vi "sensors mega.vi"() -> ()   [LabVIEW 2011]
uses:
  <vilib>/LabVIEW Interface for Arduino/Type Defs/Board Type.ctl
  <vilib>/LabVIEW Interface for Arduino/Type Defs/Pin Mode.ctl
  <vilib>/LabVIEW Interface for Arduino/Type Defs/Analog Pin.ctl
  <vilib>/LabVIEW Interface for Arduino/LabVIEW Interface for Arduino.lvlib
panel:
  in  "stop 12":bool
  out "Voltage 3":dbl(knob) scale=0.0..5.0
  out "tank":dbl(slide) scale=0.0..100.0
  out "Voltage 2":dbl(knob) scale=0.0..5.0
  out "Voltage":dbl(knob) scale=0.0..5.0
  in  "stop 11":bool
  out "Light Pos1":dbl(slide) scale=0.0..100.0
  out "Light Pos2":dbl(slide) scale=0.0..100.0
  out "Solar Pos1":bool
  out "Solar Pos2":bool
  in  "stop 10":bool
  out "Month":dbl
  in  "stop 8":bool
  in  "Wahsing Machine":bool
  in  "Dryer":bool
  in  "stop 7":bool
  in  "stop 6":bool
  in  "stop":bool
  out "Light Intensity (0 - 100) Pos2":dbl(knob) scale=0.0..100.0
  in  "stop 3":bool
  in  "stop 9":bool
  out "Water Voltage":dbl(knob) scale=0.0..5.0
  out "Low Level Water":bool
  in  "Units 2":enum16{"Celsius", "Fahrenheit", "Kelvin"}(ring)
  in  "stop 5":bool
  out "Water Temperature":dbl(slide) scale=0.0..100.0
  in  "Units":enum16{"Celsius", "Fahrenheit", "Kelvin"}(ring)
  in  "stop 4":bool
  out "Temperature Inside":dbl(slide) scale=0.0..100.0
  out "Light Intensity (0 - 100)Pos 1":dbl(knob) scale=0.0..100.0
  in  "stop 2":bool
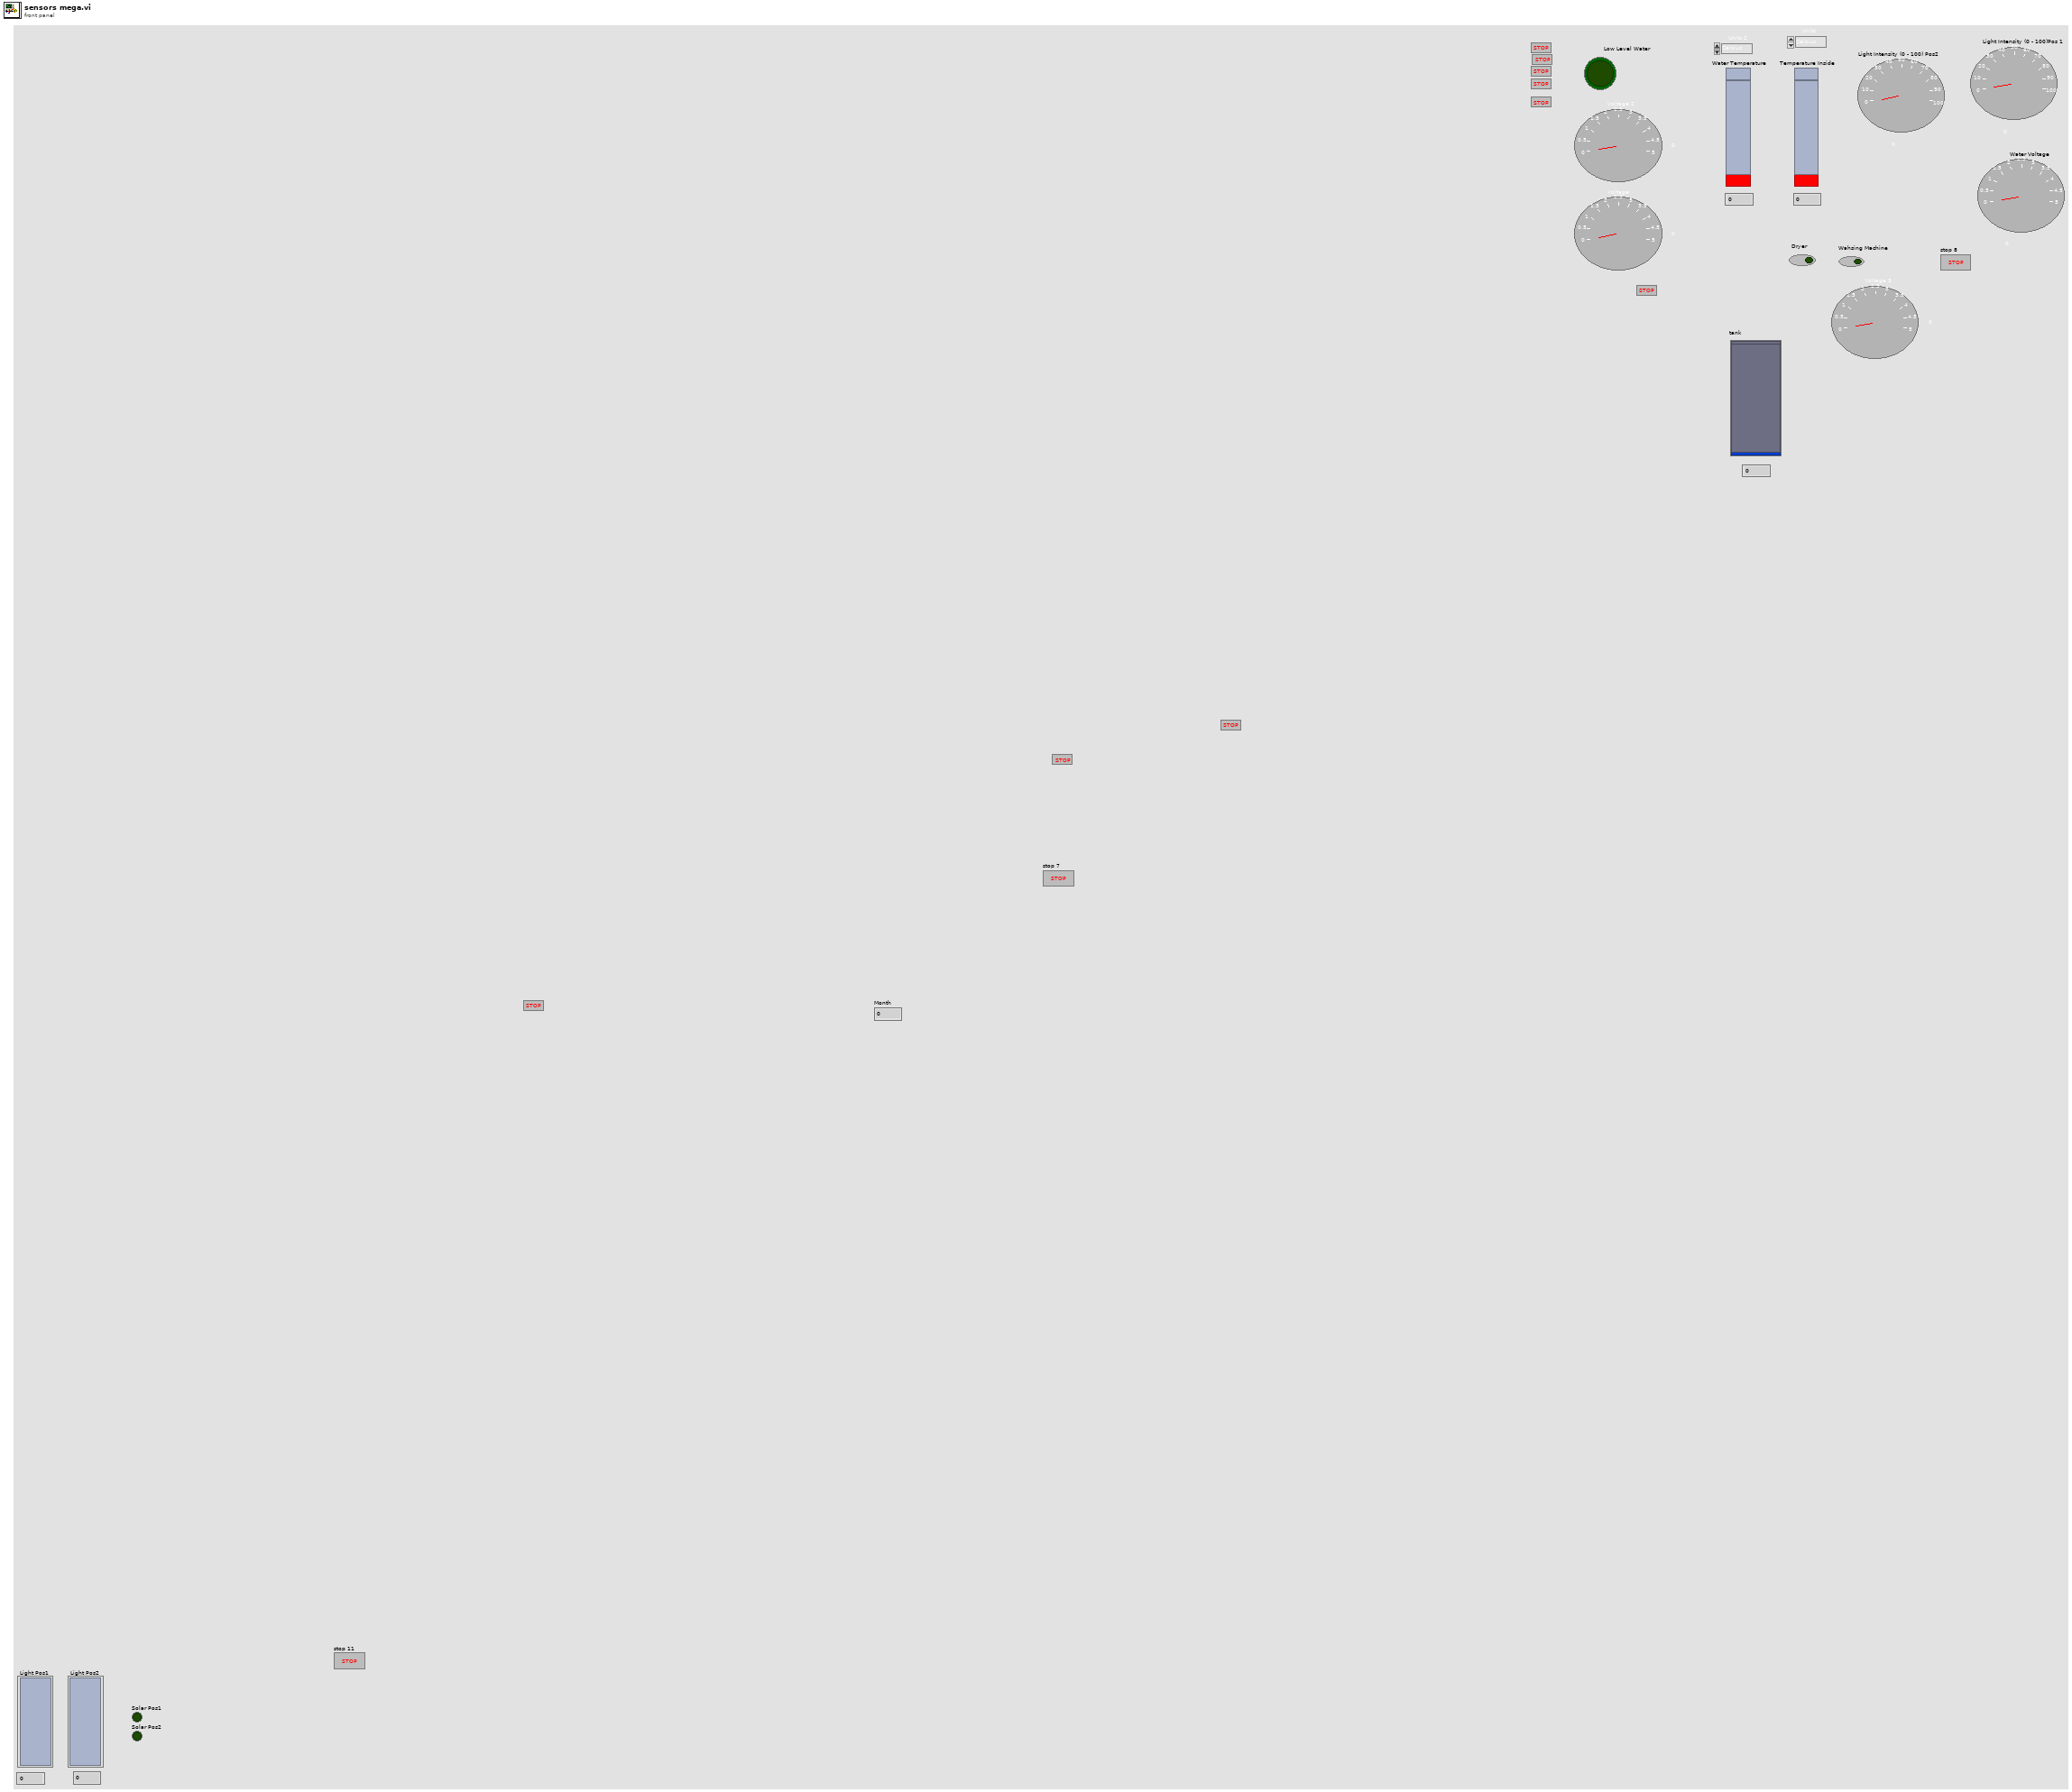
[diagram p1: front panel]
types:
  T1 = typedef "LabVIEW Interface for Arduino.lvlib/Board Type.ctl" = enum16{"Uno", "Dimuelanove w/Atmega 328", "Mega 2560"}
  T2 = typedef "LabVIEW Interface for Arduino.lvlib/Arduino Resource.ctl" = cluster{"VISA resource":refnum<visa-resource-name>, "Board Type":T1, "Connection Type":enum8{"USB / Serial"}, "Bytes Per Packet (15)":u8}
  T3 = typedef "LabVIEW Interface for Arduino.lvlib/Analog Pin.ctl" = enum8{"Anlog In 0", "Anlog In 1", "Anlog In 2", "Anlog In 3", "Anlog In 4", "Anlog In 5"}
  T4 = typedef "LabVIEW Interface for Arduino.lvlib/Pin Mode.ctl" = enum8{"Input", "Output"}
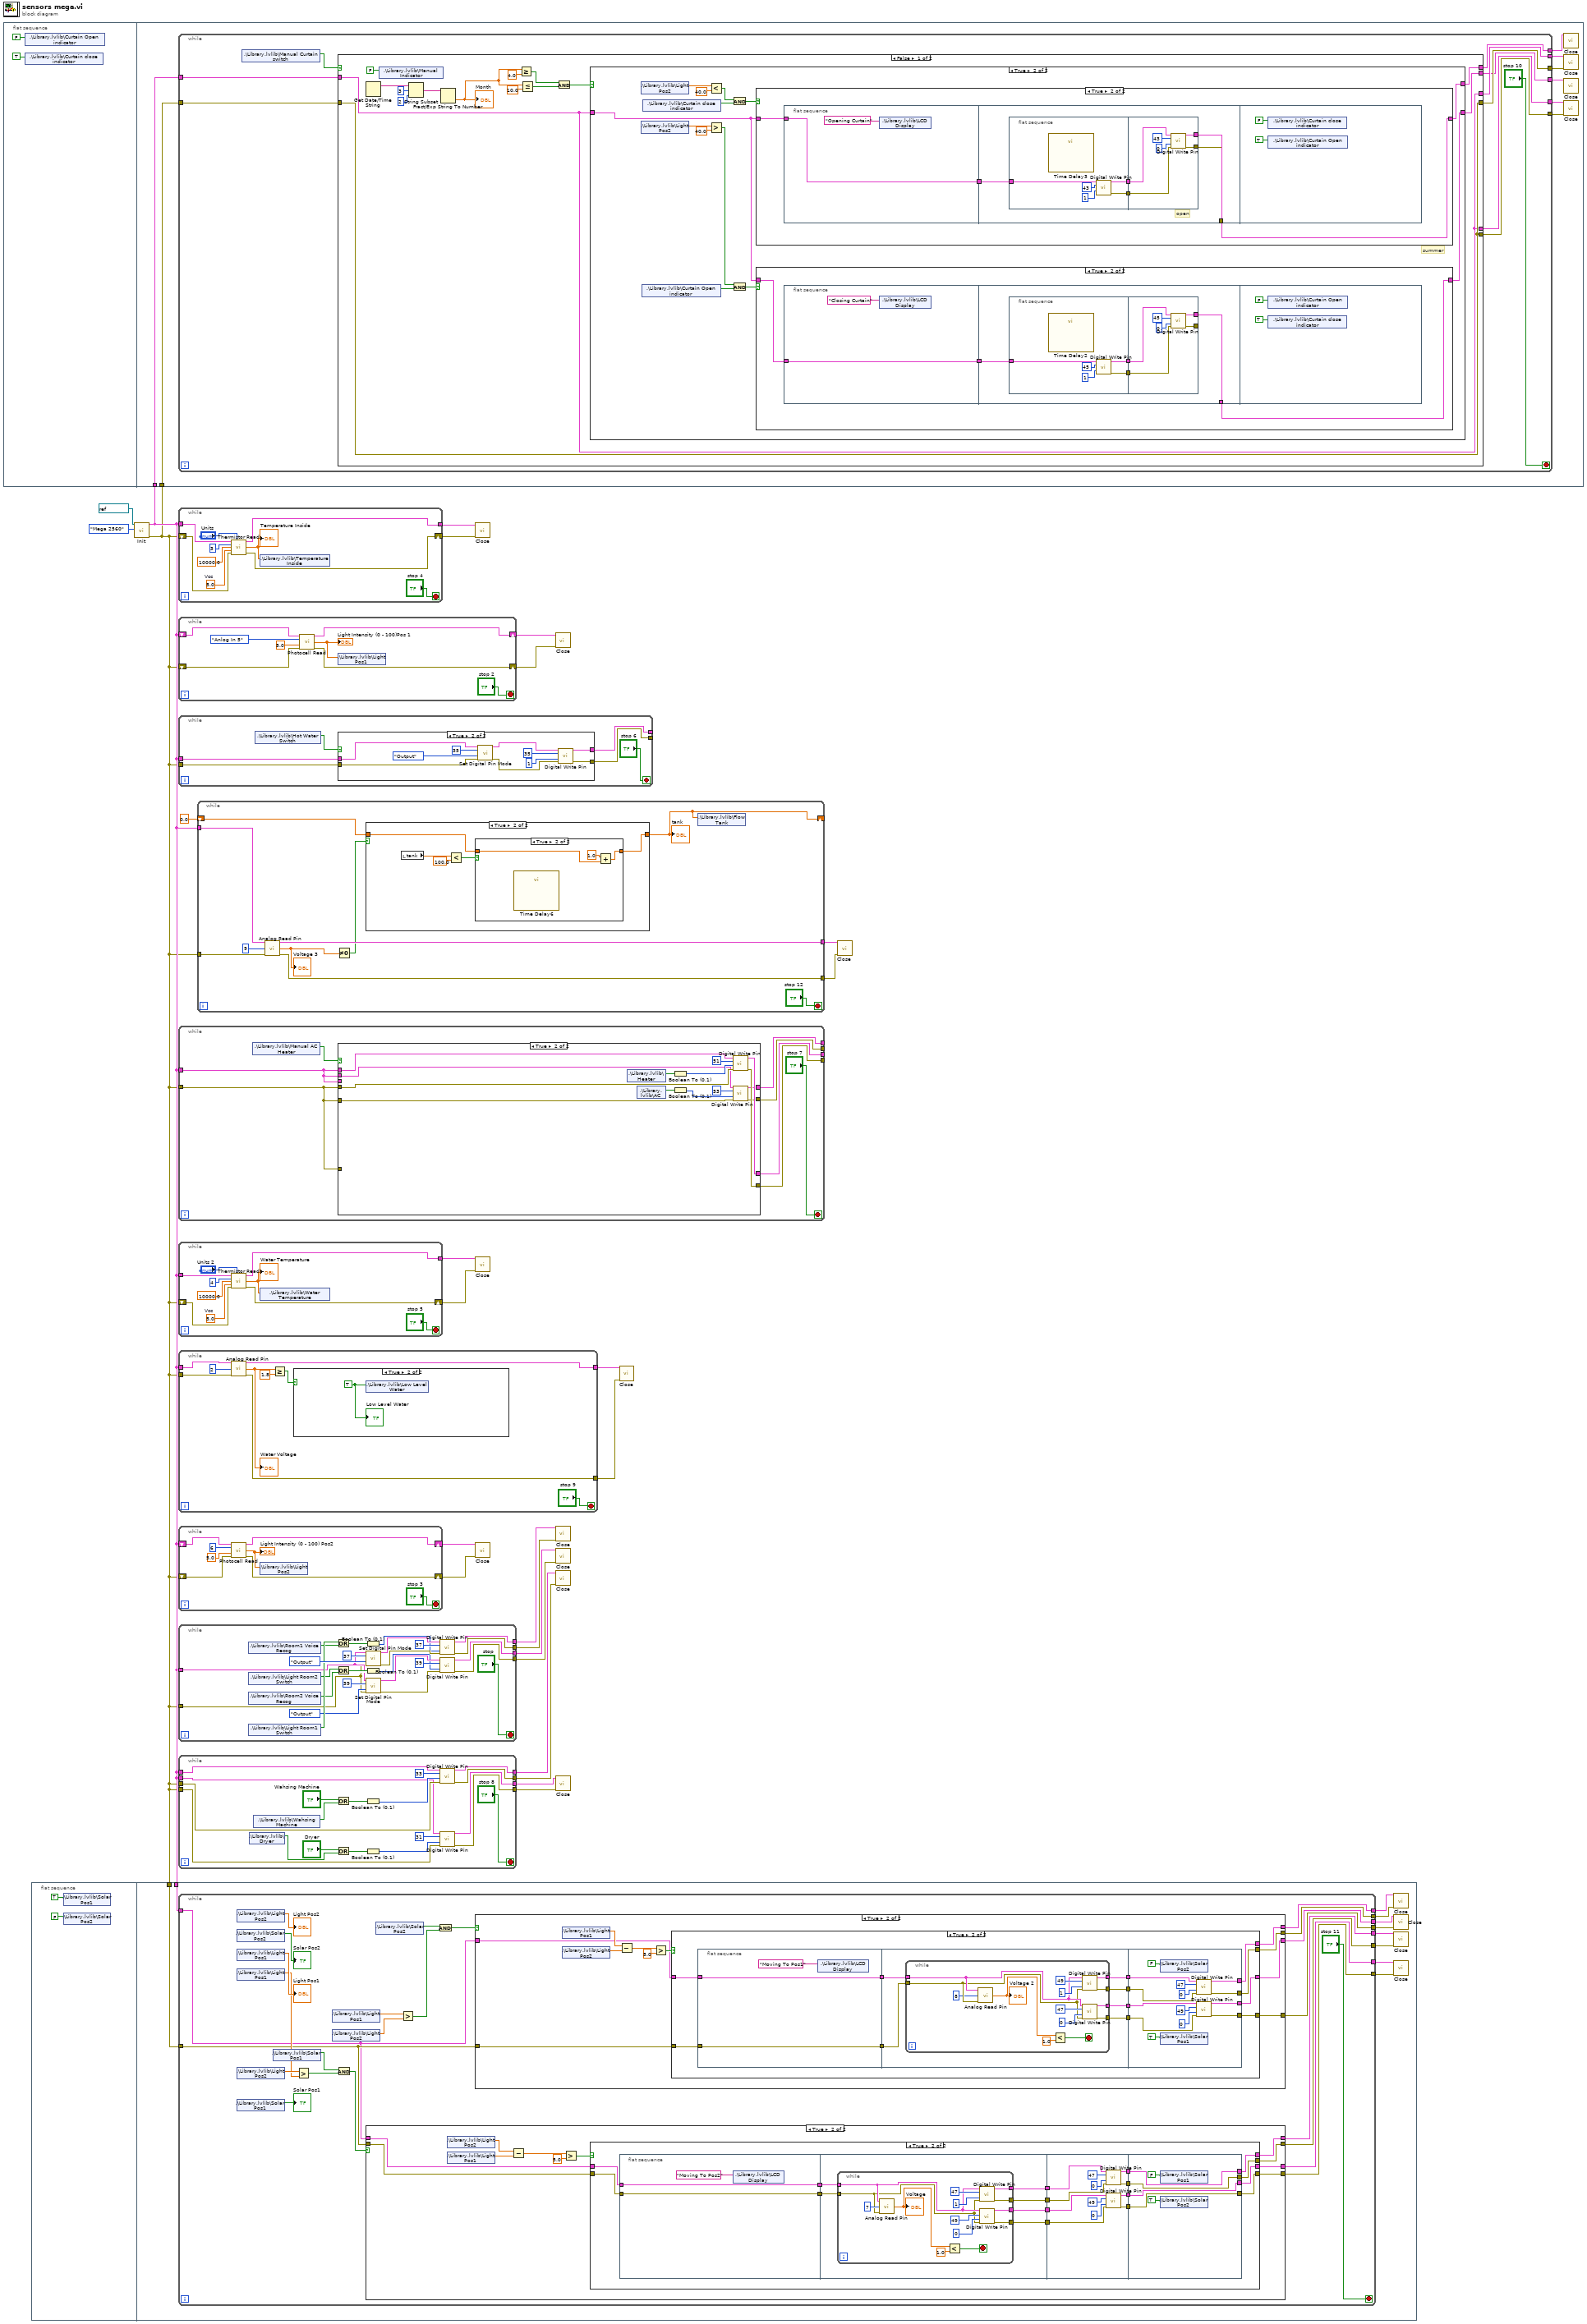
[diagram p0: block diagram]
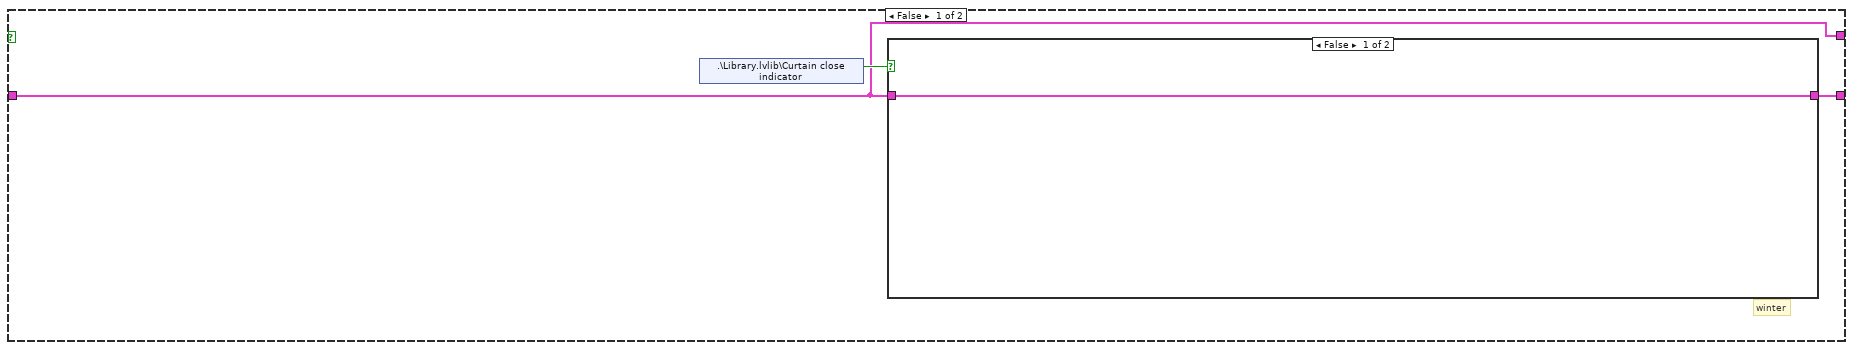
[diagram p8: hidden frame]
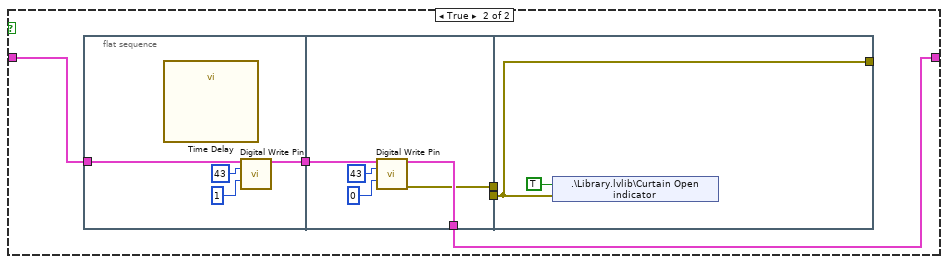
[diagram p9: hidden frame]
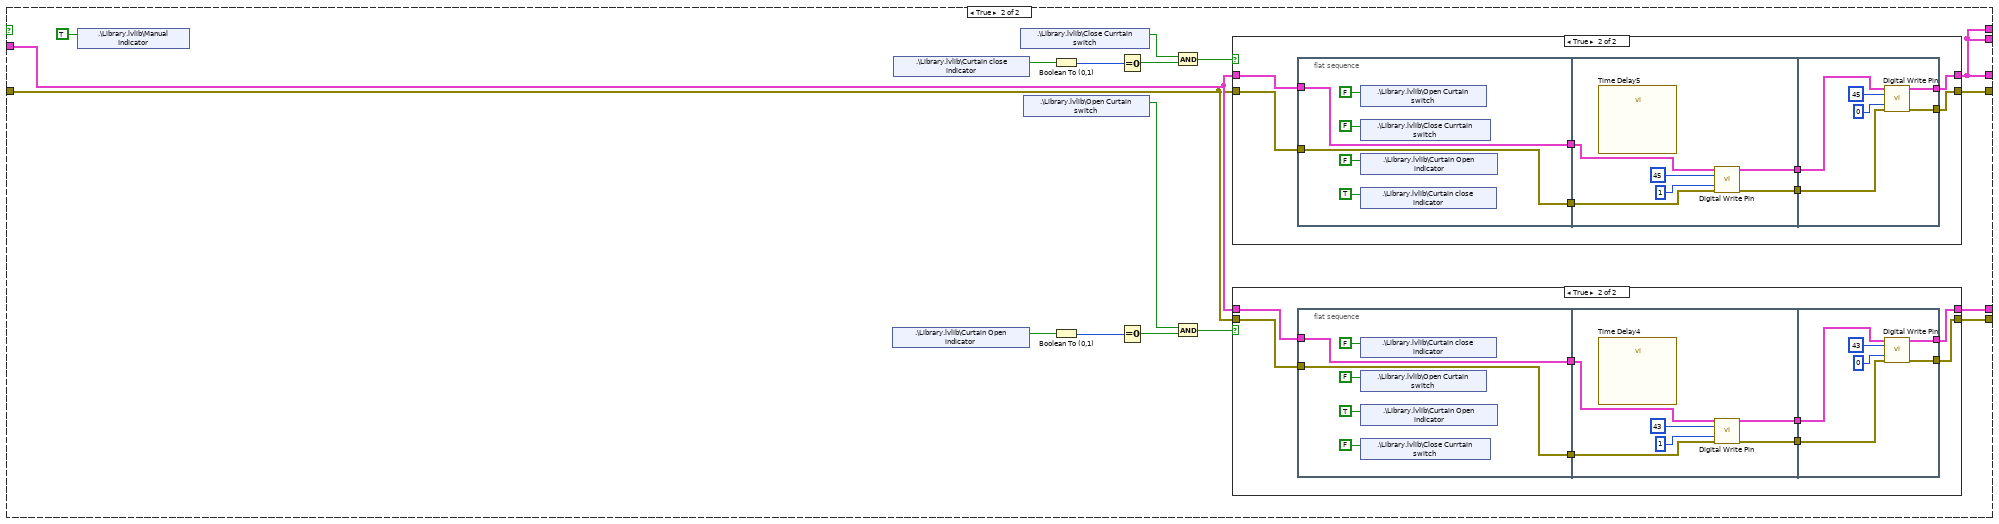
[diagram p12: hidden frame]
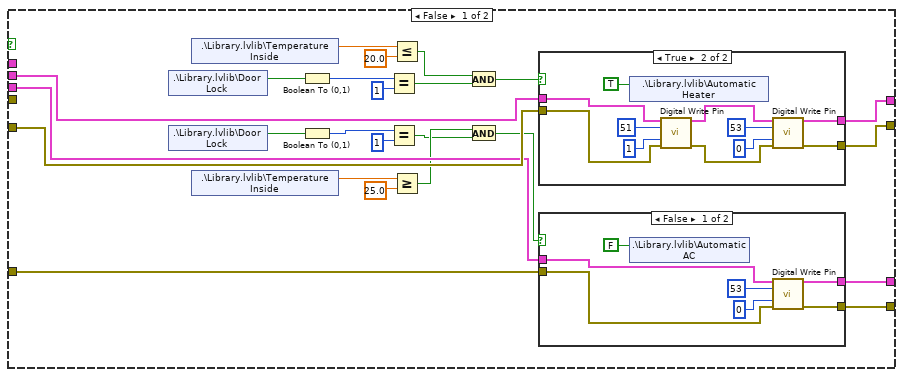
[diagram p15: hidden frame]
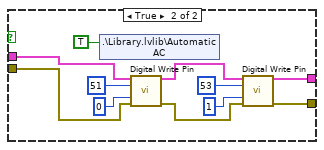
[diagram p16: hidden frame]
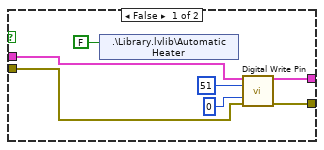
[diagram p17: hidden frame]
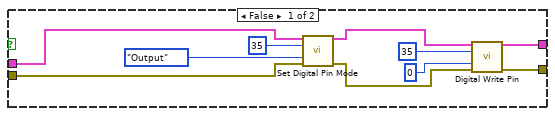
[diagram p18: hidden frame]
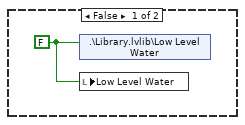
[diagram p19: hidden frame]
diagram:
  n1 = flat-sequence {
    tunnel: w2 -> [w29]
    tunnel: w1 -> [w28]
    frame #0 {
      n2 = shared-variable ".\\Library.lvlib\\Curtain Open indicator"(FALSE ("Open")) -> ()  [unwired: 1 in, 1 out]
      n3 = shared-variable ".\\Library.lvlib\\Curtain close indicator"(TRUE ("Close")) -> ()  [unwired: 1 in, 1 out]
    }
    frame #1 {
      n4 = while {
        tunnel: w29 -> [w42]
        tunnel: w28 -> [w41]
        tunnel: [w44] -> w35
        tunnel: [w43] -> w34
        tunnel: [w40] -> w33
        tunnel: [w39] -> w32
        tunnel: [w37] -> w31
        tunnel: [w36] -> w30
        stop <- "stop 10" stop-if-true
        n5 = shared-variable ".\\Library.lvlib\\Manual Curtain switch"() -> (w38:bool)  [unwired: 1 in, 1 out]
        n6 = case shown="False" w38 {
          tunnel: [w47 w156] -> w44
          tunnel: [w50 w155] -> w43
          tunnel: w42 -> [w47 w154]
          tunnel: w41 -> [w50 w153]
          tunnel: [w47 w140] -> w40
          tunnel: [w50 w152] -> w39
          tunnel: [w48 w140] -> w37
          tunnel: [w46 w140] -> w36
          frame False {
            n7 = Get Date/Time String() -> (date string=w60:string)  [unwired: 3 in, 1 out]
            n8 = shared-variable ".\\Library.lvlib\\Manual Indicator"(FALSE ("Manual Curtain switch")) -> ()  [unwired: 1 in, 1 out]
            n9 = String Subset(string=w60, offset (0)=3, length (rest)=2 ("length (rest)")) -> (substring=w57:string)
            n10 = Fract/Exp String To Number(string=w57) -> (number=w54:dbl)  [unwired: 3 in, 1 out]
            "Month" <- w54
            n11 = Greater Or Equal?(x=w54, y=4.0) -> (x >= y?=w55:bool)
            n12 = Less Or Equal?(x=w54, y=10.0) -> (x <= y?=w52:bool)
            n13 = And(x=w55, y=w52) -> (x .and. y?=w51:bool)
            n14 = case shown="True" w51 {
              tunnel: [w62 w82] -> w48
              tunnel: w47 -> [w61 w81]
              tunnel: [w61 w80] -> w46
              frame False {
                # "winter"
                n15 = shared-variable ".\\Library.lvlib\\Curtain close indicator"() -> (w63:bool)  [unwired: 1 in, 1 out]
                n16 = case shown="False" w63 {
                  tunnel: [w64 w68] -> w62
                  tunnel: w61 -> [w64 w67]
                  frame False {
                  }
                  frame True {
                    n17 = flat-sequence {
                      tunnel: w67 -> [w70]
                      tunnel: [w69] -> w66
                      tunnel: [w75] -> w68
                      tunnel: w66 -> [w74]
                      tunnel: [w73] -> w65
                      tunnel: [w79] -> _
                      tunnel: w65 -> [w79]
                      frame #0 {
                        n18 = call "Time Delay"() -> ()  [unwired: 11 in, 1 out]
                        n19 = call <vilib>:"Digital Write Pin.vi"("Arduino Resource"=w70, "Digital I/O Pin (0)"=u8 43, "Value (0)"=u8 1) -> ("Arduino Resource"=w69:T2)  [unwired: 11 in, 1 out]
                      }
                      frame #1 {
                        n20 = call <vilib>:"Digital Write Pin.vi"("Arduino Resource"=w74, "Digital I/O Pin (0)"=u8 43, "Value (0)"=u8 0) -> ("Arduino Resource"=w75:T2, "error out"=w73:errorcluster)  [unwired: 11 in]
                      }
                      frame #2 {
                        n21 = shared-variable ".\\Library.lvlib\\Curtain Open indicator"(TRUE ("Curtain Open indicator"), error in=w79) -> ()  [unwired: 1 out]
                      }
                    }
                  }
                }
              }
              frame True {
                # "summer"
                n22 = shared-variable ".\\Library.lvlib\\Light Pos2"() -> (w88:dbl)  [unwired: 1 in, 1 out]
                n23 = shared-variable ".\\Library.lvlib\\Light Pos2"() -> (w92:dbl)  [unwired: 1 in, 1 out]
                n24 = shared-variable ".\\Library.lvlib\\Curtain Open indicator"() -> (w89:bool)  [unwired: 1 in, 1 out]
                n25 = shared-variable ".\\Library.lvlib\\Curtain close indicator"() -> (w85:bool)  [unwired: 1 in, 1 out]
                n26 = Less?(x=w88, y=40.0) -> (x < y?=w86:bool)
                n27 = Greater?(x=w92, y=40.0) -> (0:w90:bool)
                n28 = And(x=w86, y=w85) -> (x .and. y?=w83:bool)
                n29 = And(x=w90, y=w89) -> (x .and. y?=w84:bool)
                n30 = case shown="True" w83 {
                  tunnel: w81 -> [w93 w96]
                  tunnel: [w93 w95] -> w80
                  frame False {
                  }
                  frame True {
                    n31 = flat-sequence {
                      tunnel: w96 -> [w98]
                      tunnel: [w98] -> w94
                      tunnel: [w100] -> w95
                      tunnel: [w99] -> _
                      tunnel: w94 -> [w101]
                      frame #0 {
                        n32 = shared-variable ".\\Library.lvlib\\LCD Display"("Opening Curtain" ("LCD Display")) -> ()  [unwired: 1 in, 1 out]
                      }
                      frame #1 {
                        # "open"
                        n33 = flat-sequence {
                          tunnel: [w105] -> w103
                          tunnel: [w104] -> w102
                          tunnel: w101 -> [w106]
                          tunnel: w103 -> [w112]
                          tunnel: w102 -> [w111]
                          tunnel: [w110] -> w100
                          tunnel: [w109] -> w99
                          frame #0 {
                            n34 = call "Time Delay3"() -> ()  [unwired: 11 in, 1 out]
                            n35 = call <vilib>:"Digital Write Pin.vi"("Arduino Resource"=w106, "Digital I/O Pin (0)"=u8 43, "Value (0)"=u8 1) -> ("Arduino Resource"=w104:T2, "error out"=w105:errorcluster)  [unwired: 11 in]
                          }
                          frame #1 {
                            n36 = call <vilib>:"Digital Write Pin.vi"("Arduino Resource"=w111, "Digital I/O Pin (0)"=u8 43, "Value (0)"=u8 0, "error in"=w112) -> ("Arduino Resource"=w110:T2, "error out"=w109:errorcluster)  [unwired: 10 in]
                          }
                        }
                      }
                      frame #2 {
                        n37 = shared-variable ".\\Library.lvlib\\Curtain close indicator"(FALSE ("Curtain close indicator")) -> ()  [unwired: 1 in, 1 out]
                        n38 = shared-variable ".\\Library.lvlib\\Curtain Open indicator"(TRUE ("Curtain Open indicator")) -> ()  [unwired: 1 in, 1 out]
                      }
                    }
                  }
                }
                n39 = case shown="True" w84 {
                  tunnel: w81 -> [w117 w120]
                  tunnel: [w117 w119] -> w82
                  frame False {
                  }
                  frame True {
                    n40 = flat-sequence {
                      tunnel: w120 -> [w122]
                      tunnel: [w122] -> w118
                      tunnel: [w123] -> w119
                      tunnel: w118 -> [w124]
                      frame #0 {
                        n41 = shared-variable ".\\Library.lvlib\\LCD Display"("Closing Curtain" ("LCD Display")) -> ()  [unwired: 1 in, 1 out]
                      }
                      frame #1 {
                        n42 = flat-sequence {
                          tunnel: [w129] -> w126
                          tunnel: [w128] -> w125
                          tunnel: w124 -> [w127]
                          tunnel: w126 -> [w135]
                          tunnel: w125 -> [w134]
                          tunnel: [w133] -> w123
                          tunnel: [w132] -> _
                          frame #0 {
                            n43 = call "Time Delay2"() -> ()  [unwired: 11 in, 1 out]
                            n44 = call <vilib>:"Digital Write Pin.vi"("Arduino Resource"=w127, "Digital I/O Pin (0)"=u8 45, "Value (0)"=u8 1) -> ("Arduino Resource"=w128:T2, "error out"=w129:errorcluster)  [unwired: 11 in]
                          }
                          frame #1 {
                            n45 = call <vilib>:"Digital Write Pin.vi"("Arduino Resource"=w134, "Digital I/O Pin (0)"=u8 45, "Value (0)"=u8 0, "error in"=w135) -> ("Arduino Resource"=w133:T2, "error out"=w132:errorcluster)  [unwired: 10 in]
                          }
                        }
                      }
                      frame #2 {
                        n46 = shared-variable ".\\Library.lvlib\\Curtain Open indicator"(FALSE ("Curtain Open indicator")) -> ()  [unwired: 1 in, 1 out]
                        n47 = shared-variable ".\\Library.lvlib\\Curtain close indicator"(TRUE ("Curtain close indicator")) -> ()  [unwired: 1 in, 1 out]
                      }
                    }
                  }
                }
              }
            }
          }
          frame True {
            n48 = shared-variable ".\\Library.lvlib\\Manual Indicator"(TRUE ("Manual Curtain")) -> ()  [unwired: 1 in, 1 out]
            n49 = shared-variable ".\\Library.lvlib\\Curtain Open indicator"() -> (w141:bool)  [unwired: 1 in, 1 out]
            n50 = shared-variable ".\\Library.lvlib\\Curtain close indicator"() -> (w142:bool)  [unwired: 1 in, 1 out]
            n51 = shared-variable ".\\Library.lvlib\\Close Currtain switch"() -> (w144:bool)  [unwired: 1 in, 1 out]
            n52 = shared-variable ".\\Library.lvlib\\Open Curtain switch"() -> (w145:bool)  [unwired: 1 in, 1 out]
            n53 = Boolean To (0,1)(Boolean=w142) -> (0, 1=w148:i16)
            n54 = Boolean To (0,1)(Boolean=w141) -> (0, 1=w151:i16)
            n55 = Equal To 0?(x=w148) -> (x = 0?=w149:bool)
            n56 = Equal To 0?(x=w151) -> (x = 0?=w150:bool)
            n57 = And(x=w144, y=w149) -> (x .and. y?=w147:bool)
            n58 = And(x=w145, y=w150) -> (x .and. y?=w146:bool)
            n59 = case shown="True" w147 {
              tunnel: w154 -> [w158 w166]
              tunnel: w153 -> [w157 w165]
              tunnel: [w158 w162] -> w140
              tunnel: [w157 w161] -> w152
              frame False {
              }
              frame True {
                n60 = flat-sequence {
                  tunnel: w165 -> [w171]
                  tunnel: w166 -> [w172]
                  tunnel: [w172] -> w160
                  tunnel: [w171] -> w159
                  tunnel: [w174] -> w164
                  tunnel: [w173] -> w163
                  tunnel: w160 -> [w176]
                  tunnel: w159 -> [w175]
                  tunnel: w164 -> [w182]
                  tunnel: w163 -> [w181]
                  tunnel: [w180] -> w162
                  tunnel: [w179] -> w161
                  frame #0 {
                    n61 = shared-variable ".\\Library.lvlib\\Open Curtain switch"(FALSE ("Close Currtain switch")) -> ()  [unwired: 1 in, 1 out]
                    n62 = shared-variable ".\\Library.lvlib\\Close Currtain switch"(FALSE ("Close Currtain switch")) -> ()  [unwired: 1 in, 1 out]
                    n63 = shared-variable ".\\Library.lvlib\\Curtain Open indicator"(FALSE ("Open")) -> ()  [unwired: 1 in, 1 out]
                    n64 = shared-variable ".\\Library.lvlib\\Curtain close indicator"(TRUE ("Open")) -> ()  [unwired: 1 in, 1 out]
                  }
                  frame #1 {
                    n65 = call "Time Delay5"() -> ()  [unwired: 11 in, 1 out]
                    n66 = call <vilib>:"Digital Write Pin.vi"("Arduino Resource"=w176, "Digital I/O Pin (0)"=u8 45, "Value (0)"=u8 1, "error in"=w175) -> ("Arduino Resource"=w173:T2, "error out"=w174:errorcluster)  [unwired: 10 in]
                  }
                  frame #2 {
                    n67 = call <vilib>:"Digital Write Pin.vi"("Arduino Resource"=w181, "Digital I/O Pin (0)"=u8 45, "Value (0)"=u8 0, "error in"=w182) -> ("Arduino Resource"=w180:T2, "error out"=w179:errorcluster)  [unwired: 10 in]
                  }
                }
              }
            }
            n68 = case shown="True" w146 {
              tunnel: w154 -> [w186 w194]
              tunnel: w153 -> [w185 w193]
              tunnel: [w186 w190] -> w156
              tunnel: [w185 w189] -> w155
              frame False {
              }
              frame True {
                n69 = flat-sequence {
                  tunnel: w193 -> [w199]
                  tunnel: w194 -> [w200]
                  tunnel: [w200] -> w188
                  tunnel: [w199] -> w187
                  tunnel: [w202] -> w192
                  tunnel: [w201] -> w191
                  tunnel: w188 -> [w204]
                  tunnel: w187 -> [w203]
                  tunnel: w192 -> [w210]
                  tunnel: w191 -> [w209]
                  tunnel: [w208] -> w190
                  tunnel: [w207] -> w189
                  frame #0 {
                    n70 = shared-variable ".\\Library.lvlib\\Curtain close indicator"(FALSE ("Open")) -> ()  [unwired: 1 in, 1 out]
                    n71 = shared-variable ".\\Library.lvlib\\Open Curtain switch"(FALSE ("Close Currtain switch")) -> ()  [unwired: 1 in, 1 out]
                    n72 = shared-variable ".\\Library.lvlib\\Curtain Open indicator"(TRUE ("Open")) -> ()  [unwired: 1 in, 1 out]
                    n73 = shared-variable ".\\Library.lvlib\\Close Currtain switch"(FALSE ("Close Currtain switch")) -> ()  [unwired: 1 in, 1 out]
                  }
                  frame #1 {
                    n74 = call "Time Delay4"() -> ()  [unwired: 11 in, 1 out]
                    n75 = call <vilib>:"Digital Write Pin.vi"("Arduino Resource"=w204, "Digital I/O Pin (0)"=u8 43, "Value (0)"=u8 1, "error in"=w203) -> ("Arduino Resource"=w201:T2, "error out"=w202:errorcluster)  [unwired: 10 in]
                  }
                  frame #2 {
                    n76 = call <vilib>:"Digital Write Pin.vi"("Arduino Resource"=w209, "Digital I/O Pin (0)"=u8 43, "Value (0)"=u8 0, "error in"=w210) -> ("Arduino Resource"=w208:T2, "error out"=w207:errorcluster)  [unwired: 10 in]
                  }
                }
              }
            }
          }
        }
      }
      n77 = call <vilib>:"Close.vi"("Arduino Resource"=w30) -> ()  [unwired: 14 in, 1 out]
      n78 = call <vilib>:"Close.vi"("Arduino Resource"=w33, "error in"=w32) -> ()  [unwired: 13 in, 1 out]
      n79 = call <vilib>:"Close.vi"("Arduino Resource"=w31) -> ()  [unwired: 14 in, 1 out]
      n80 = call <vilib>:"Close.vi"("Arduino Resource"=w35, "error in"=w34) -> ()  [unwired: 13 in, 1 out]
    }
  }
  n81 = flat-sequence {
    tunnel: w2 -> [w216]
    tunnel: w1 -> [w215]
    frame #0 {
      n82 = shared-variable ".\\Library.lvlib\\Solar Pos1"(TRUE ("Solar Pos1")) -> ()  [unwired: 1 in, 1 out]
      n83 = shared-variable ".\\Library.lvlib\\Solar Pos2"(FALSE ("Solar Pos2")) -> ()  [unwired: 1 in, 1 out]
    }
    frame #1 {
      n84 = while {
        tunnel: w216 -> [w225]
        tunnel: w215 -> [w230]
        tunnel: [w241] -> w224
        tunnel: [w240] -> w223
        tunnel: [w239] -> w222
        tunnel: [w238] -> w221
        tunnel: [w234] -> w220
        tunnel: [w233] -> w219
        tunnel: [w232] -> w218
        tunnel: [w231] -> w217
        stop <- "stop 11" stop-if-true
        n85 = shared-variable ".\\Library.lvlib\\Light Pos2"() -> (→"Light Pos2":dbl)  [unwired: 1 in, 1 out]
        n86 = shared-variable ".\\Library.lvlib\\Solar Pos2"() -> (→"Solar Pos2":bool)  [unwired: 1 in, 1 out]
        n87 = shared-variable ".\\Library.lvlib\\Light Pos1"() -> (→"Light Pos1":dbl)  [unwired: 1 in, 1 out]
        n88 = shared-variable ".\\Library.lvlib\\Light Pos1"() -> (w244:dbl)  [unwired: 1 in, 1 out]
        n89 = shared-variable ".\\Library.lvlib\\Light Pos2"() -> (w245:dbl)  [unwired: 1 in, 1 out]
        n90 = shared-variable ".\\Library.lvlib\\Solar Pos1"() -> (→"Solar Pos1":bool)  [unwired: 1 in, 1 out]
        n91 = shared-variable ".\\Library.lvlib\\Solar Pos1"() -> (w246:bool)  [unwired: 1 in, 1 out]
        n92 = Greater?(x=w245, y=w244) -> (0:w243:bool)
        n93 = shared-variable ".\\Library.lvlib\\Light Pos1"() -> (w229:dbl)  [unwired: 1 in, 1 out]
        n94 = shared-variable ".\\Library.lvlib\\Light Pos2"() -> (w228:dbl)  [unwired: 1 in, 1 out]
        n95 = And(x=w246, y=w243) -> (x .and. y?=w242:bool)
        n96 = case shown="True" w242 {
          tunnel: w225 -> [w315 w321]
          tunnel: w230 -> [w314 w320]
          tunnel: [w315 w319] -> w241
          tunnel: [w314 w318] -> w240
          tunnel: [w315 w317] -> w239
          tunnel: [w314 w316] -> w238
          frame False {
          }
          frame True {
            n97 = shared-variable ".\\Library.lvlib\\Light Pos2"() -> (w326:dbl)  [unwired: 1 in, 1 out]
            n98 = shared-variable ".\\Library.lvlib\\Light Pos1"() -> (w325:dbl)  [unwired: 1 in, 1 out]
            n99 = Subtract(x=w326, y=w325) -> (x-y=w323:dbl)
            n100 = Greater?(x=w323, y=5.0) -> (0:w324:bool)
            n101 = case shown="True" w324 {
              tunnel: w321 -> [w328 w344]
              tunnel: w320 -> [w327 w343]
              tunnel: [w328 w338] -> w319
              tunnel: [w327 w337] -> w318
              tunnel: [w328 w336] -> w317
              tunnel: [w327 w335] -> w316
              frame False {
              }
              frame True {
                n102 = flat-sequence {
                  tunnel: w343 -> [w346]
                  tunnel: w344 -> [w347]
                  tunnel: [w347] -> w330
                  tunnel: [w346] -> w329
                  tunnel: [w351] -> w342
                  tunnel: [w350] -> w341
                  tunnel: [w349] -> w340
                  tunnel: [w348] -> w339
                  tunnel: w330 -> [w353]
                  tunnel: w329 -> [w352]
                  tunnel: w342 -> [w376]
                  tunnel: w341 -> [w375]
                  tunnel: w340 -> [w374]
                  tunnel: w339 -> [w372]
                  tunnel: [w371] -> w334
                  tunnel: [w370] -> w333
                  tunnel: [w369] -> w332
                  tunnel: [w368] -> w331
                  tunnel: [w382] -> w335
                  tunnel: [w383] -> w336
                  tunnel: [w384] -> w337
                  tunnel: [w385] -> w338
                  tunnel: w334 -> [w385]
                  tunnel: w333 -> [w384]
                  tunnel: w332 -> [w383]
                  tunnel: w331 -> [w382]
                  frame #0 {
                    n103 = shared-variable ".\\Library.lvlib\\LCD Display"("Moving To Pos2" ("LCD Display")) -> ()  [unwired: 1 in, 1 out]
                  }
                  frame #1 {
                    n104 = while {
                      tunnel: w353 -> [w356]
                      tunnel: w352 -> [w355]
                      tunnel: [w363] -> w351
                      tunnel: [w362] -> w350
                      tunnel: [w361] -> w349
                      tunnel: [w360] -> w348
                      stop <- w354 stop-if-true
                      n105 = call <vilib>:"Analog Read Pin.vi"("Arduino Resource"=w356, "Analog Input Pin (0)"=u8 7, "error in"=w355) -> ("Voltage"=w358:dbl)  [unwired: 10 in, 2 out]
                      "Voltage" <- w358
                      n106 = Less?(x=w358, y=1.0) -> (x < y?=w354:bool)
                      n107 = call <vilib>:"Digital Write Pin.vi"("Arduino Resource"=w356, "Digital I/O Pin (0)"=u8 47, "Value (0)"=u8 1, "error in"=w355) -> ("Arduino Resource"=w363:T2, "error out"=w362:errorcluster)  [unwired: 10 in]
                      n108 = call <vilib>:"Digital Write Pin.vi"("Arduino Resource"=w356, "Digital I/O Pin (0)"=u8 49, "Value (0)"=u8 0, "error in"=w355) -> ("Arduino Resource"=w361:T2, "error out"=w360:errorcluster)  [unwired: 10 in]
                    }
                  }
                  frame #2 {
                    n109 = call <vilib>:"Digital Write Pin.vi"("Arduino Resource"=w376, "Digital I/O Pin (0)"=u8 47, "Value (0)"=u8 0, "error in"=w375) -> ("Arduino Resource"=w371:T2, "error out"=w370:errorcluster)  [unwired: 10 in]
                    n110 = call <vilib>:"Digital Write Pin.vi"("Arduino Resource"=w374, "Digital I/O Pin (0)"=u8 49, "Value (0)"=u8 0, "error in"=w372) -> ("Arduino Resource"=w369:T2, "error out"=w368:errorcluster)  [unwired: 10 in]
                  }
                  frame #3 {
                    n111 = shared-variable ".\\Library.lvlib\\Solar Pos1"(FALSE ("Solar Pos1")) -> ()  [unwired: 1 in, 1 out]
                    n112 = shared-variable ".\\Library.lvlib\\Solar Pos2"(TRUE ("Solar Pos2")) -> ()  [unwired: 1 in, 1 out]
                  }
                }
              }
            }
          }
        }
        n113 = shared-variable ".\\Library.lvlib\\Solar Pos2"() -> (w235:bool)  [unwired: 1 in, 1 out]
        n114 = Greater?(x=w229, y=w228) -> (0:w236:bool)
        n115 = And(x=w235, y=w236) -> (x .and. y?=w237:bool)
        n116 = case shown="True" w237 {
          tunnel: w225 -> [w251 w257]
          tunnel: w230 -> [w250 w256]
          tunnel: [w251 w255] -> w232
          tunnel: [w250 w254] -> w231
          tunnel: [w251 w253] -> w234
          tunnel: [w250 w252] -> w233
          frame False {
          }
          frame True {
            n117 = shared-variable ".\\Library.lvlib\\Light Pos1"() -> (w262:dbl)  [unwired: 1 in, 1 out]
            n118 = shared-variable ".\\Library.lvlib\\Light Pos2"() -> (w261:dbl)  [unwired: 1 in, 1 out]
            n119 = Subtract(x=w262, y=w261) -> (x-y=w259:dbl)
            n120 = Greater?(x=w259, y=5.0) -> (0:w260:bool)
            n121 = case shown="True" w260 {
              tunnel: w257 -> [w264 w276]
              tunnel: w256 -> [w263 w275]
              tunnel: [w264 w270] -> w255
              tunnel: [w263 w269] -> w254
              tunnel: [w264 w268] -> w253
              tunnel: [w263 w267] -> w252
              frame False {
              }
              frame True {
                n122 = flat-sequence {
                  tunnel: w275 -> [w278]
                  tunnel: w276 -> [w279]
                  tunnel: [w279] -> w266
                  tunnel: [w278] -> w265
                  tunnel: [w283] -> w274
                  tunnel: [w282] -> w273
                  tunnel: [w281] -> w272
                  tunnel: [w280] -> w271
                  tunnel: w266 -> [w285]
                  tunnel: w265 -> [w284]
                  tunnel: w274 -> [w310]
                  tunnel: w273 -> [w309]
                  tunnel: w272 -> [w308]
                  tunnel: w271 -> [w306]
                  tunnel: [w305] -> w270
                  tunnel: [w304] -> w269
                  tunnel: [w303] -> w268
                  tunnel: [w302] -> w267
                  frame #0 {
                    n123 = shared-variable ".\\Library.lvlib\\LCD Display"("Moving To Pos1" ("LCD Display")) -> ()  [unwired: 1 in, 1 out]
                  }
                  frame #1 {
                    n124 = while {
                      tunnel: w285 -> [w291]
                      tunnel: w284 -> [w290]
                      tunnel: [w295] -> w283
                      tunnel: [w294] -> w282
                      tunnel: [w293] -> w281
                      tunnel: [w292] -> w280
                      stop <- w286 stop-if-true
                      n125 = call <vilib>:"Analog Read Pin.vi"("Arduino Resource"=w291, "Analog Input Pin (0)"=u8 8, "error in"=w290) -> ("Voltage"=w288:dbl)  [unwired: 10 in, 2 out]
                      "Voltage 2" <- w288
                      n126 = Less?(x=w288, y=1.0) -> (x < y?=w286:bool)
                      n127 = call <vilib>:"Digital Write Pin.vi"("Arduino Resource"=w291, "Digital I/O Pin (0)"=u8 49, "Value (0)"=u8 1, "error in"=w290) -> ("Arduino Resource"=w295:T2, "error out"=w294:errorcluster)  [unwired: 10 in]
                      n128 = call <vilib>:"Digital Write Pin.vi"("Arduino Resource"=w291, "Digital I/O Pin (0)"=u8 47, "Value (0)"=u8 0, "error in"=w290) -> ("Arduino Resource"=w293:T2, "error out"=w292:errorcluster)  [unwired: 10 in]
                    }
                  }
                  frame #2 {
                    n129 = shared-variable ".\\Library.lvlib\\Solar Pos2"(FALSE ("Solar Pos2")) -> ()  [unwired: 1 in, 1 out]
                    n130 = shared-variable ".\\Library.lvlib\\Solar Pos1"(TRUE ("Solar Pos1")) -> ()  [unwired: 1 in, 1 out]
                    n131 = call <vilib>:"Digital Write Pin.vi"("Arduino Resource"=w310, "Digital I/O Pin (0)"=u8 47, "Value (0)"=u8 0, "error in"=w309) -> ("Arduino Resource"=w305:T2, "error out"=w304:errorcluster)  [unwired: 10 in]
                    n132 = call <vilib>:"Digital Write Pin.vi"("Arduino Resource"=w308, "Digital I/O Pin (0)"=u8 49, "Value (0)"=u8 0, "error in"=w306) -> ("Arduino Resource"=w303:T2, "error out"=w302:errorcluster)  [unwired: 10 in]
                  }
                }
              }
            }
          }
        }
      }
      n133 = call <vilib>:"Close.vi"("Arduino Resource"=w218, "error in"=w217) -> ()  [unwired: 13 in, 1 out]
      n134 = call <vilib>:"Close.vi"("Arduino Resource"=w220, "error in"=w219) -> ()  [unwired: 13 in, 1 out]
      n135 = call <vilib>:"Close.vi"("Arduino Resource"=w224, "error in"=w223) -> ()  [unwired: 13 in, 1 out]
      n136 = call <vilib>:"Close.vi"("Arduino Resource"=w222, "error in"=w221) -> ()  [unwired: 13 in, 1 out]
    }
  }
  n137 = call <vilib>:"Init.vi"("VISA resource"=refnum<visa-resource-name> "COM4", "Board Type (Uno)"=Board_Type."Mega 2560") -> ("Arduino Resource"=w2:T2, "error out"=w1:errorcluster)  [unwired: 16 in]
  n138 = while {
    tunnel: w2 -> [w395]
    shift-right: [w393] -> w20
    shift-left: w1 -> [w394]
    tunnel: [w392] -> w21
    stop <- "stop 4" stop-if-true
    w391 = 5.0  # Vcc
    n139 = call <vilib>:"Thermistor Read.vi"("Arduino Resource"=w395, "Units (C)"="Units", "Thermistor AI Pin (0)"=u8 3 ("Thermistor AI Pin"), "Paired Resistance (10K Ohms)"=10000.0 ("Paired Resistance (Ohms)"), "Vcc (5 v)"=w391, "error in"=w394) -> ("Arduino Resource"=w392:T2, "Temperature"=w386:dbl, "error out"=w393:errorcluster)  [unwired: 7 in]
    "Temperature Inside" <- w386
    n140 = shared-variable ".\\Library.lvlib\\Temperature Inside"(w386) -> ()  [unwired: 1 in, 1 out]
  }
  n141 = while {
    shift-right: [w400] -> w22
    shift-left: w1 -> [w403]
    shift-right: [w402] -> w23
    shift-left: w2 -> [w399]
    stop <- "stop 2" stop-if-true
    n142 = call <vilib>:"Photocell Read.vi"("Arduino Resource"=w399, "Photo Cell Pin (0)"=Analog_Pin."Anlog In 5" ("Photo Cell Pin (AI 0-5)"), "Vcc (5)"=5.0 ("Vcc"), "error in"=w403) -> ("Arduino Resource"=w402:T2, "Light Intensity (0 - 100)"=w396:dbl, "error out"=w400:errorcluster)  [unwired: 9 in]
    "Light Intensity (0 - 100)Pos 1" <- w396
    n143 = shared-variable ".\\Library.lvlib\\Light Pos1"(w396) -> ()  [unwired: 1 in, 1 out]
  }
  n144 = while {
    tunnel: w2 -> [w405]
    tunnel: w1 -> [w404]
    tunnel: [w407] -> _
    tunnel: [w406] -> _
    stop <- "stop 6" stop-if-true
    n145 = shared-variable ".\\Library.lvlib\\Hot Water Switch"() -> (w408:bool)  [unwired: 1 in, 1 out]
    n146 = case shown="True" w408 {
      tunnel: [w412 w429] -> w407
      tunnel: [w411 w428] -> w406
      tunnel: w405 -> [w414 w427]
      tunnel: w404 -> [w413 w426]
      frame False {
        n147 = call <vilib>:"Set Digital Pin Mode.vi"("Arduino Resource"=w414, "Digital I/O Pin"=u8 35, "Pin Mode (Input)"=Pin_Mode."Output", "error in"=w413) -> ("Arduino Resource"=w419:T2, "error out"=w418:errorcluster)  [unwired: 10 in]
        n148 = call <vilib>:"Digital Write Pin.vi"("Arduino Resource"=w419, "Digital I/O Pin (0)"=u8 35, "Value (0)"=u8 0, "error in"=w418) -> ("Arduino Resource"=w412:T2, "error out"=w411:errorcluster)  [unwired: 10 in]
      }
      frame True {
        n149 = call <vilib>:"Set Digital Pin Mode.vi"("Arduino Resource"=w427, "Digital I/O Pin"=u8 35, "Pin Mode (Input)"=Pin_Mode."Output", "error in"=w426) -> ("Arduino Resource"=w425:T2, "error out"=w424:errorcluster)  [unwired: 10 in]
        n150 = call <vilib>:"Digital Write Pin.vi"("Arduino Resource"=w425, "Digital I/O Pin (0)"=u8 35, "Value (0)"=u8 1, "error in"=w424) -> ("Arduino Resource"=w429:T2, "error out"=w428:errorcluster)  [unwired: 10 in]
      }
    }
  }
  n151 = while {
    tunnel: [w436] -> _
    tunnel: [w435] -> _
    tunnel: w2 -> [w431]
    tunnel: w1 -> [w430]
    tunnel: [w433] -> _
    tunnel: [w434] -> _
    stop <- "stop 7" stop-if-true
    n152 = shared-variable ".\\Library.lvlib\\Manual AC Heater"() -> (w432:bool)  [unwired: 1 in, 1 out]
    n153 = case shown="True" w432 {
      tunnel: w431 -> [_ w511]
      tunnel: w430 -> [_ w510]
      tunnel: [w451 w508] -> w436
      tunnel: [w450 w507] -> w435
      tunnel: [w456 w504] -> w434
      tunnel: [w457 w503] -> w433
      tunnel: w430 -> [w458 w501]
      tunnel: w431 -> [w459 w500]
      tunnel: w431 -> [w453 _]
      tunnel: w430 -> [w452 _]
      frame False {
        n154 = shared-variable ".\\Library.lvlib\\Door Lock"() -> (w448:bool)  [unwired: 1 in, 1 out]
        n155 = shared-variable ".\\Library.lvlib\\Door Lock"() -> (w444:bool)  [unwired: 1 in, 1 out]
        n156 = shared-variable ".\\Library.lvlib\\Temperature Inside"() -> (w461:dbl)  [unwired: 1 in, 1 out]
        n157 = shared-variable ".\\Library.lvlib\\Temperature Inside"() -> (w454:dbl)  [unwired: 1 in, 1 out]
        n158 = Boolean To (0,1)(Boolean=w448) -> (0, 1=w440:i16)
        n159 = Boolean To (0,1)(Boolean=w444) -> (0, 1=w442:i16)
        n160 = Equal?(x=w440, y=i16 1) -> (x = y?=w438:bool)
        n161 = Equal?(x=w442, y=i16 1) -> (x = y?=w443:bool)
        n162 = Less Or Equal?(x=w461, y=20.0) -> (x <= y?=w449:bool)
        n163 = Greater Or Equal?(x=w454, y=25.0) -> (x >= y?=w447:bool)
        n164 = And(x=w449, y=w438) -> (x .and. y?=w445:bool)
        n165 = And(x=w447, y=w443) -> (x .and. y?=w446:bool)
        n166 = case shown="True" w445 {
          tunnel: w459 -> [w486 w493]
          tunnel: w458 -> [w483 w492]
          tunnel: [w485 w489] -> w457
          tunnel: [w484 w488] -> w456
          frame False {
            n167 = shared-variable ".\\Library.lvlib\\Automatic Heater"(FALSE ("Automatic AC")) -> ()  [unwired: 1 in, 1 out]
            n168 = call <vilib>:"Digital Write Pin.vi"("Arduino Resource"=w486, "Digital I/O Pin (0)"=u8 51, "Value (0)"=u8 0, "error in"=w483) -> ("Arduino Resource"=w485:T2, "error out"=w484:errorcluster)  [unwired: 10 in]
          }
          frame True {
            n169 = shared-variable ".\\Library.lvlib\\Automatic Heater"(TRUE ("Automatic AC")) -> ()  [unwired: 1 in, 1 out]
            n170 = call <vilib>:"Digital Write Pin.vi"("Arduino Resource"=w493, "Digital I/O Pin (0)"=u8 51, "Value (0)"=u8 1, "error in"=w492) -> ("Arduino Resource"=w491:T2, "error out"=w490:errorcluster)  [unwired: 10 in]
            n171 = call <vilib>:"Digital Write Pin.vi"("Arduino Resource"=w491, "Digital I/O Pin (0)"=u8 53, "Value (0)"=u8 0, "error in"=w490) -> ("Arduino Resource"=w489:T2, "error out"=w488:errorcluster)  [unwired: 10 in]
          }
        }
        n172 = case shown="False" w446 {
          tunnel: w453 -> [w464 w475]
          tunnel: w452 -> [w466 w474]
          tunnel: [w463 w471] -> w451
          tunnel: [w465 w470] -> w450
          frame False {
            n173 = shared-variable ".\\Library.lvlib\\Automatic AC"(FALSE ("Automatic AC")) -> ()  [unwired: 1 in, 1 out]
            n174 = call <vilib>:"Digital Write Pin.vi"("Arduino Resource"=w464, "Digital I/O Pin (0)"=u8 53, "Value (0)"=u8 0, "error in"=w466) -> ("Arduino Resource"=w463:T2, "error out"=w465:errorcluster)  [unwired: 10 in]
          }
          frame True {
            n175 = shared-variable ".\\Library.lvlib\\Automatic AC"(TRUE ("Automatic AC")) -> ()  [unwired: 1 in, 1 out]
            n176 = call <vilib>:"Digital Write Pin.vi"("Arduino Resource"=w475, "Digital I/O Pin (0)"=u8 51, "Value (0)"=u8 0, "error in"=w474) -> ("Arduino Resource"=w473:T2, "error out"=w472:errorcluster)  [unwired: 10 in]
            n177 = call <vilib>:"Digital Write Pin.vi"("Arduino Resource"=w473, "Digital I/O Pin (0)"=u8 53, "Value (0)"=u8 1, "error in"=w472) -> ("Arduino Resource"=w471:T2, "error out"=w470:errorcluster)  [unwired: 10 in]
          }
        }
      }
      frame True {
        n178 = shared-variable ".\\Library.lvlib\\Heater"() -> (w498:bool)  [unwired: 1 in, 1 out]
        n179 = shared-variable ".\\Library.lvlib\\AC"() -> (w499:bool)  [unwired: 1 in, 1 out]
        n180 = Boolean To (0,1)(Boolean=w498) -> (0, 1=w506:i16)
        n181 = Boolean To (0,1)(Boolean=w499) -> (0, 1=w505:i16)
        n182 = call <vilib>:"Digital Write Pin.vi"("Arduino Resource"=w511, "Digital I/O Pin (0)"=u8 51, "Value (0)"=w506, "error in"=w510) -> ("Arduino Resource"=w508:T2, "error out"=w507:errorcluster)  [unwired: 10 in]
        n183 = call <vilib>:"Digital Write Pin.vi"("Arduino Resource"=w500, "Digital I/O Pin (0)"=u8 53, "Value (0)"=w505, "error in"=w501) -> ("Arduino Resource"=w503:T2, "error out"=w504:errorcluster)  [unwired: 10 in]
      }
    }
  }
  n184 = while {
    tunnel: w2 -> [w521]
    shift-right: [w519] -> w18
    shift-left: w1 -> [w520]
    tunnel: [w518] -> w19
    stop <- "stop 5" stop-if-true
    w517 = 5.0  # Vcc
    n185 = call <vilib>:"Thermistor Read.vi"("Arduino Resource"=w521, "Units (C)"="Units 2", "Thermistor AI Pin (0)"=u8 4 ("Thermistor AI Pin"), "Paired Resistance (10K Ohms)"=10000.0 ("Paired Resistance (Ohms)"), "Vcc (5 v)"=w517, "error in"=w520) -> ("Arduino Resource"=w518:T2, "Temperature"=w512:dbl, "error out"=w519:errorcluster)  [unwired: 7 in]
    "Water Temperature" <- w512
    n186 = shared-variable ".\\Library.lvlib\\Water Temperature"(w512) -> ()  [unwired: 1 in, 1 out]
  }
  n187 = while {
    tunnel: w2 -> [w529]
    tunnel: w1 -> [w528]
    tunnel: [w526] -> w17
    tunnel: [w525] -> w16
    stop <- "stop 9" stop-if-true
    n188 = call <vilib>:"Analog Read Pin.vi"("Arduino Resource"=w529, "Analog Input Pin (0)"=u8 2, "error in"=w528) -> ("Arduino Resource"=w526:T2, "Voltage"=w524:dbl, "error out"=w525:errorcluster)  [unwired: 10 in]
    "Water Voltage" <- w524
    n189 = Greater Or Equal?(x=w524, y=1.8) -> (x >= y?=w522:bool)
    n190 = case shown="True" w522 {
      frame False {
        w531 = FALSE ("Low Level Water")
        n191 = shared-variable ".\\Library.lvlib\\Low Level Water"(w531) -> ()  [unwired: 1 in, 1 out]
        n192 = local write "Low Level Water"(w531) -> ()
      }
      frame True {
        w532 = TRUE ("Low Level Water")
        n193 = shared-variable ".\\Library.lvlib\\Low Level Water"(w532) -> ()  [unwired: 1 in, 1 out]
        "Low Level Water" <- w532
      }
    }
  }
  n194 = while {
    shift-right: [w537] -> w14
    shift-left: w1 -> [w540]
    shift-right: [w539] -> w15
    shift-left: w2 -> [w536]
    stop <- "stop 3" stop-if-true
    n195 = call <vilib>:"Photocell Read.vi"("Arduino Resource"=w536, "Photo Cell Pin (0)"=u8 6, "Vcc (5)"=5.0 ("Vcc"), "error in"=w540) -> ("Arduino Resource"=w539:T2, "Light Intensity (0 - 100)"=w534:dbl, "error out"=w537:errorcluster)  [unwired: 9 in]
    "Light Intensity (0 - 100) Pos2" <- w534
    n196 = shared-variable ".\\Library.lvlib\\Light Pos2"(w534) -> ()  [unwired: 1 in, 1 out]
  }
  n197 = while {
    tunnel: w2 -> [w544]
    tunnel: w1 -> [w543]
    tunnel: [w564] -> w13
    tunnel: [w563] -> w12
    tunnel: [w542] -> w11
    tunnel: [w541] -> w10
    stop <- "stop" stop-if-true
    n198 = shared-variable ".\\Library.lvlib\\Room1 Voice Recog"() -> (w555:bool)  [unwired: 1 in, 1 out]
    n199 = shared-variable ".\\Library.lvlib\\Light Room2 Switch"() -> (w546:bool)  [unwired: 1 in, 1 out]
    n200 = shared-variable ".\\Library.lvlib\\Room2 Voice Recog"() -> (w547:bool)  [unwired: 1 in, 1 out]
    n201 = shared-variable ".\\Library.lvlib\\Light Room1 Switch"() -> (w556:bool)  [unwired: 1 in, 1 out]
    n202 = Or(x=w556, y=w555) -> (x .or. y?=w554:bool)
    n203 = Or(x=w546, y=w547) -> (x .or. y?=w545:bool)
    n204 = Boolean To (0,1)(Boolean=w554) -> (0, 1=w557:i16)
    n205 = Boolean To (0,1)(Boolean=w545) -> (0, 1=w548:i16)
    n206 = call <vilib>:"Set Digital Pin Mode.vi"("Arduino Resource"=w544, "Digital I/O Pin"=u8 37, "Pin Mode (Input)"=Pin_Mode."Output", "error in"=w543) -> ("Arduino Resource"=w562:T2, "error out"=w561:errorcluster)  [unwired: 10 in]
    n207 = call <vilib>:"Set Digital Pin Mode.vi"("Arduino Resource"=w544, "Digital I/O Pin"=u8 39, "Pin Mode (Input)"=Pin_Mode."Output", "error in"=w543) -> ("Arduino Resource"=w553:T2, "error out"=w552:errorcluster)  [unwired: 10 in]
    n208 = call <vilib>:"Digital Write Pin.vi"("Arduino Resource"=w562, "Digital I/O Pin (0)"=u8 37, "Value (0)"=w557, "error in"=w561) -> ("Arduino Resource"=w564:T2, "error out"=w563:errorcluster)  [unwired: 10 in]
    n209 = call <vilib>:"Digital Write Pin.vi"("Arduino Resource"=w553, "Digital I/O Pin (0)"=u8 39, "Value (0)"=w548, "error in"=w552) -> ("Arduino Resource"=w542:T2, "error out"=w541:errorcluster)  [unwired: 10 in]
  }
  n210 = while {
    tunnel: w2 -> [w583]
    tunnel: w1 -> [w582]
    tunnel: [w580] -> w9
    tunnel: [w579] -> w8
    tunnel: w2 -> [w572]
    tunnel: w1 -> [w573]
    tunnel: [w575] -> w6
    tunnel: [w576] -> w7
    stop <- "stop 8" stop-if-true
    n211 = shared-variable ".\\Library.lvlib\\Dryer"() -> (w569:bool)  [unwired: 1 in, 1 out]
    n212 = shared-variable ".\\Library.lvlib\\Wahsing Machine"() -> (w566:bool)  [unwired: 1 in, 1 out]
    n213 = Or(x="Wahsing Machine", y=w566) -> (x .or. y?=w568:bool)
    n214 = Or(x="Dryer", y=w569) -> (x .or. y?=w570:bool)
    n215 = Boolean To (0,1)(Boolean=w568) -> (0, 1=w578:i16)
    n216 = Boolean To (0,1)(Boolean=w570) -> (0, 1=w577:i16)
    n217 = call <vilib>:"Digital Write Pin.vi"("Arduino Resource"=w583, "Digital I/O Pin (0)"=u8 33, "Value (0)"=w578, "error in"=w582) -> ("Arduino Resource"=w580:T2, "error out"=w579:errorcluster)  [unwired: 10 in]
    n218 = call <vilib>:"Digital Write Pin.vi"("Arduino Resource"=w572, "Digital I/O Pin (0)"=u8 31, "Value (0)"=w577, "error in"=w573) -> ("Arduino Resource"=w575:T2, "error out"=w576:errorcluster)  [unwired: 10 in]
  }
  n219 = while {
    tunnel: w2 -> [w593]
    tunnel: [w592] -> w5
    tunnel: w1 -> [w591]
    tunnel: [w589] -> w4
    shift-right: [w585] -> _
    shift-left: 0.0 -> [w586]
    stop <- "stop 12" stop-if-true
    n220 = call <vilib>:"Analog Read Pin.vi"("Arduino Resource"=w593, "Analog Input Pin (0)"=u8 9, "error in"=w591) -> ("Arduino Resource"=w592:T2, "Voltage"=w588:dbl, "error out"=w589:errorcluster)  [unwired: 10 in]
    "Voltage 3" <- w588
    n221 = Not Equal To 0?(x=w588) -> (x != 0?=w587:bool)
    n222 = case shown="True" w587 {
      tunnel: w586 -> [w595 w599]
      tunnel: [w595 w600] -> w585
      frame False {
      }
      frame True {
        n223 = local read "tank"() -> (w598:dbl)
        n224 = Less?(x=w598, y=100.0) -> (x < y?=w596:bool)
        n225 = case shown="True" w596 {
          tunnel: [w601 w603] -> w600
          tunnel: w599 -> [w601 w602]
          frame False {
          }
          frame True {
            n226 = call "Time Delay6"() -> ()  [unwired: 11 in, 1 out]
            n227 = Add(x=1.0, y=w602) -> (x+y=w603:dbl)
          }
        }
      }
    }
    "tank" <- w585
    n228 = shared-variable ".\\Library.lvlib\\Flow Tank"(w585) -> ()  [unwired: 1 in, 1 out]
  }
  n229 = call <vilib>:"Close.vi"("Arduino Resource"=w21, "error in"=w20) -> ()  [unwired: 13 in, 1 out]
  n230 = call <vilib>:"Close.vi"("Arduino Resource"=w19, "error in"=w18) -> ()  [unwired: 13 in, 1 out]
  n231 = call <vilib>:"Close.vi"("Arduino Resource"=w15, "error in"=w14) -> ()  [unwired: 13 in, 1 out]
  n232 = call <vilib>:"Close.vi"("Arduino Resource"=w23, "error in"=w22) -> ()  [unwired: 13 in, 1 out]
  n233 = call <vilib>:"Close.vi"("Arduino Resource"=w13, "error in"=w12) -> ()  [unwired: 13 in, 1 out]
  n234 = call <vilib>:"Close.vi"("Arduino Resource"=w11, "error in"=w10) -> ()  [unwired: 13 in, 1 out]
  n235 = call <vilib>:"Close.vi"("Arduino Resource"=w9, "error in"=w8) -> ()  [unwired: 13 in, 1 out]
  n236 = call <vilib>:"Close.vi"("Arduino Resource"=w6, "error in"=w7) -> ()  [unwired: 13 in, 1 out]
  n237 = call <vilib>:"Close.vi"("Arduino Resource"=w17, "error in"=w16) -> ()  [unwired: 13 in, 1 out]
  n238 = call <vilib>:"Close.vi"("Arduino Resource"=w5, "error in"=w4) -> ()  [unwired: 13 in, 1 out]
